vi "EventLoop 1.vi"   [LabVIEW 2017]
uses:
  Communication/Communication.lvlib
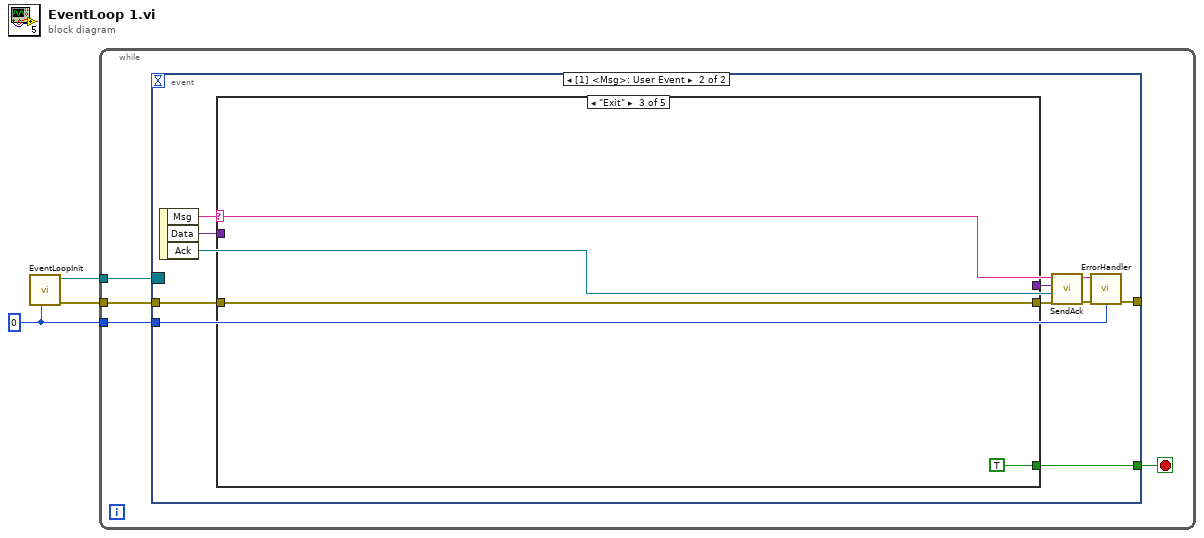
[diagram p0: block diagram]
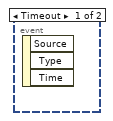
[diagram p2: hidden frame]
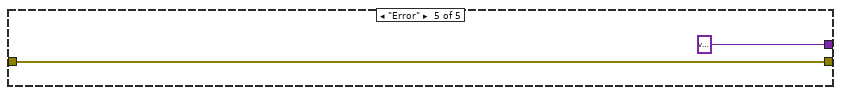
[diagram p6: hidden frame]
diagram:
  w1 = 0 ("Instance")
  n1 = call "EventLoopInit.vi"("Instance"=w1) -> ("error out"=w2:errorcluster, "Event Registration Refnum"=w3:refnum<event-registration>)  [unwired: 8 in, 1 out]
  n2 = while {
    tunnel: w3 -> [w7]
    tunnel: w2 -> [w6]
    tunnel: w1 -> [w5]
    stop <- w4 stop-if-true
    n3 = event shown="[1] <Msg>: User Event" {
      selector: w7 -> [_ _]
      dyn-events: _ -> [_ _]
      timeout: _ -> [_ _]
      tunnel: w6 -> [_ w16]
      tunnel: [_ w12] -> _
      tunnel: w5 -> [_ w11]
      tunnel: [_ w8] -> w4
      event Timeout {
        n4 = event-data() -> ()  [unwired: 1 in, 3 out]
      }
      event User Event {
        n5 = event-data() -> ("Msg"=w13:string, "Data"=w17:variant, "Ack"=w15:refnum<notifier>)  [unwired: 1 in]
        n6 = case shown="\"Exit\"" w13 {
          tunnel: w17 -> [_ _ _ _ _]
          tunnel: w16 -> [w18 w19 w21 w22 w23]
          tunnel: [_ _ _ _ variant] -> w10
          tunnel: [w18 w19 w21 w22 w23] -> w9
          tunnel: [_ _ TRUE _ _] -> w8
          frame Default {
          }
          frame "Init" {
          }
          frame "Exit" {
          }
          frame "Tick" {
          }
          frame "Error" {
          }
        }
        n7 = call "SendAck.vi"("error in (no error)"=w9, "Ack"=w15, "Variant"=w10) -> ("error out"=w14:errorcluster)  [unwired: 8 in]
        n8 = call "ErrorHandler.vi"("Instance"=w11, "error in (no error)"=w14, "Msg"=w13) -> ("error out"=w12:errorcluster)  [unwired: 8 in]
      }
    }
  }
